vi "Vision Processing old.vi"(5 "IP Addr":string="USB 0", 7 "LED Color":T3={"Hue"={35.13837107340087, 168.7186808723669}, "Sat"={139.64285714285714, 255.0}, "Val"={145.71428571428572, 255.0}} {"Hue" scale=0.0..255.0 scale format="%#_3g"}, 8 "error in (no error)":errorcluster, 11 "Image Size":T1=enum."160x120") -> ()   [LabVIEW 2015]
uses:
  Vision Support Code/Camera Types.ctl
  <vilib>/Rock Robotics/WPI/Camera/WPI_CameraImageSize.ctl
  <vilib>/Rock Robotics/WPI/Camera/WPI_CameraWhite Balance Values.ctl
  <vilib>/Rock Robotics/WPI/Camera/WPI_CameraExposure Values.ctl
  <vilib>/Rock Robotics/WPI/Camera/WPI_CameraFrameRate.ctl
  Robot Global Data.vi
  <vilib>/Rock Robotics/Network Tables/NT Write String.vi
  <vilib>/vision/NI_Vision_Development_Module.lvlib
  Vision Target Values.vi
panel:
  out "Timings":cluster{"Call Name":string, "Delta (ms)":u32}[](array[cluster])
  out "Highest Avg Score":dbl
  in  "Min Score Threshold":i32=75
  in  "Display Original":bool=TRUE
  in  "Display Mask":bool=TRUE
  out "fps":dbl
  in  "Emphasize Limit Tests":bool=TRUE
  in  "Camera Type":T2=enum."MS HD3000 square"
  in  "Aspect Fudge Factor":dbl=1.0
  in  "Score Threshold":dbl=75.0
  out "ms to process":u32
  out "Qualified Particles":i32
  # "This is only the initial camera size.\nOther camera setup is done\non the diagram. Notice it is set\nonce before the loop but can be\nupdated within the loop if needed."
  # "Instructions:\nUse LED Color to threshold and build particles. Adjust calibration if needed.\nDisplays are very useful for debugging, but will slow down execution, so you\nmay want to disable once working.\nAnnotations show the rectangle and the scores from top to bottom.\nChange camera setting on diagram."
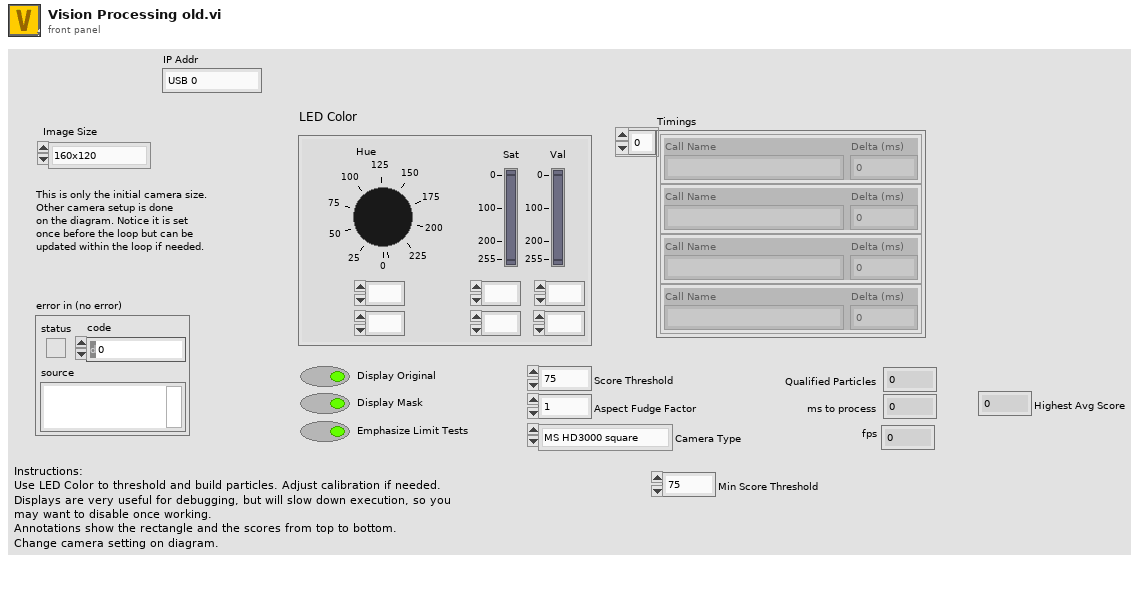
[diagram p1: front panel]
types:
  T1 = typedef "WPI_CameraImageSize.ctl" = enum16{"640x480", "320x240", "160x120", "Custom"}
  T2 = typedef "Camera Types.ctl" = enum16{"206", "1011", "1013", "MS HD3000 square", "MS HD3000 640x480"}
  T3 = cluster{"Hue":cluster{dbl, dbl}, "Sat":cluster{dbl, dbl}, "Val":cluster{dbl, dbl}}
  T4 = typedef "WPI_CameraFrameRate.ctl" = u32
  T5 = typedef "WPI_CameraExposure Values.ctl" = enum16{"Auto", "Flicker-free 50 Hz", "Flicker-free 60 Hz", "Hold current", "Custom"}
  T6 = typedef "WPI_CameraWhite Balance Values.ctl" = enum16{"Auto", "Fixed indoor", "Fixed outdoor 1", "Fixed outdoor 2", "Fixed fluorescent 1", "Fixed fluorescent 2", "Hold current", "Custom"}
  T7 = typedef "Image Type" = u32
  T8 = typedef "Particle Parameters" = i32
  T9 = typedef "WPI_CameraDevRef.ctl" = cluster{"Camera Address":string, "CameraStatus":errorcluster}
  T10 = typedef "IMAQ Image.ctl" = refnum<image>
  T11 = cluster{"Bounding box":cluster{"left":dbl, "top":dbl, "right":dbl, "bottom":dbl}, "Aspect Ratio":dbl, "Area to CH":dbl, "X Mask":dbl, "Y Mask":dbl, "Moment":dbl}[]
  T12 = cluster{"Distance (ft)":dbl, "Center":cluster{dbl, dbl}, "Normalized Rect":cluster{"Numeric":dbl, "Numeric 2":dbl, "Numeric 3":dbl, "Numeric 5":dbl}}[]
  T13 = cluster{"Detected Targets":cluster{"Distance (ft)":dbl, "Center":cluster{"X":dbl, "Y":dbl}, "Normalized Rect":cluster{"Numeric":dbl, "Numeric 2":dbl, "Numeric 3":dbl, "Numeric 5":dbl}}[]}
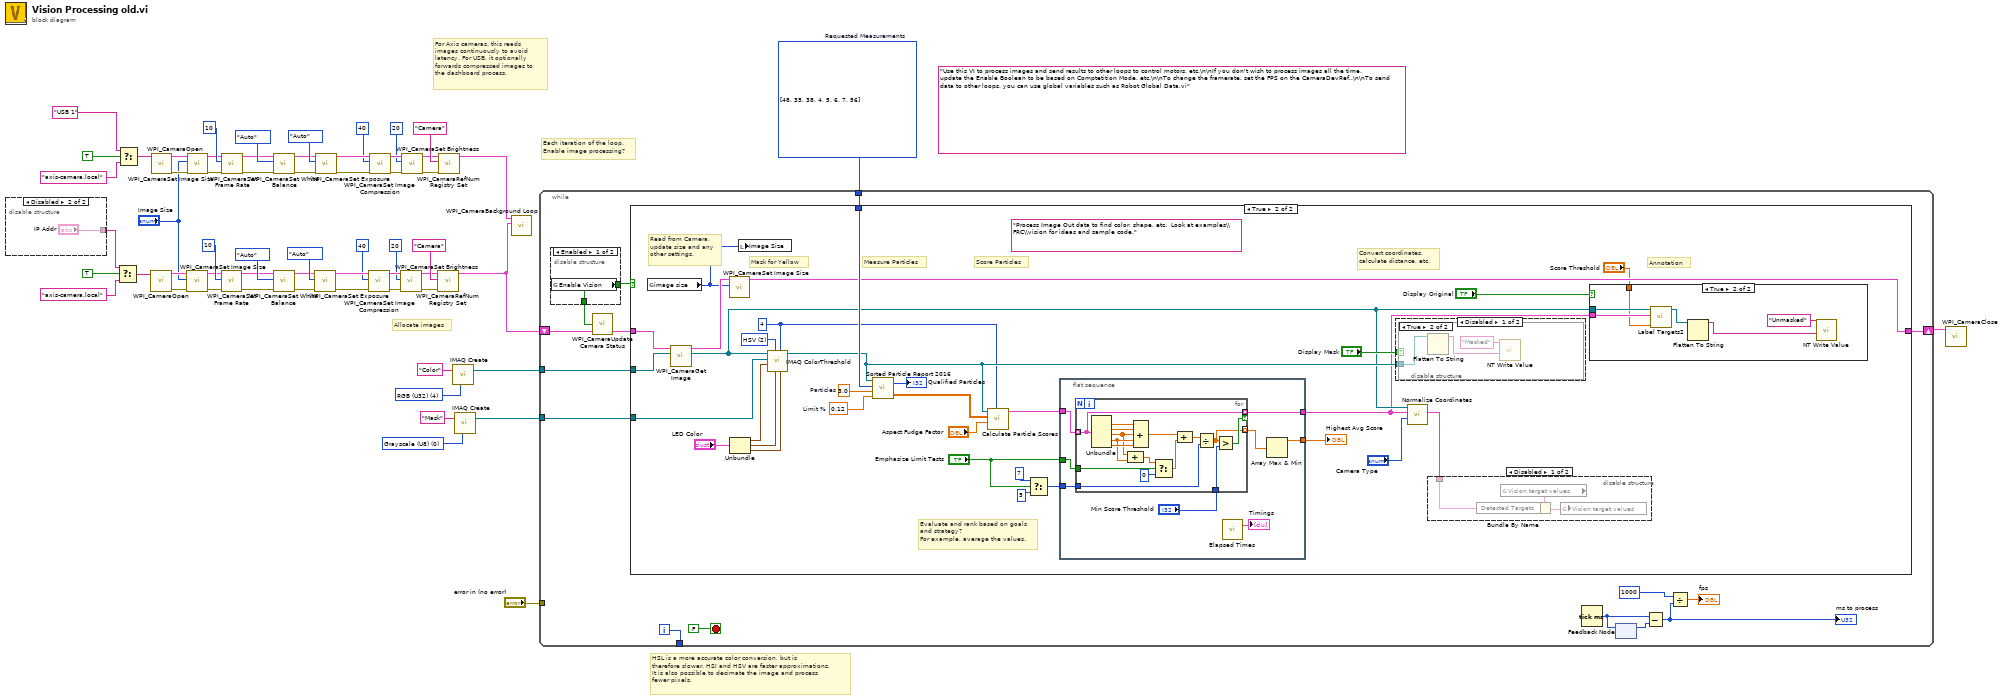
[diagram p0: block diagram]
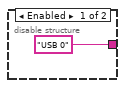
[diagram p2: hidden frame]
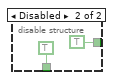
[diagram p3: hidden frame]
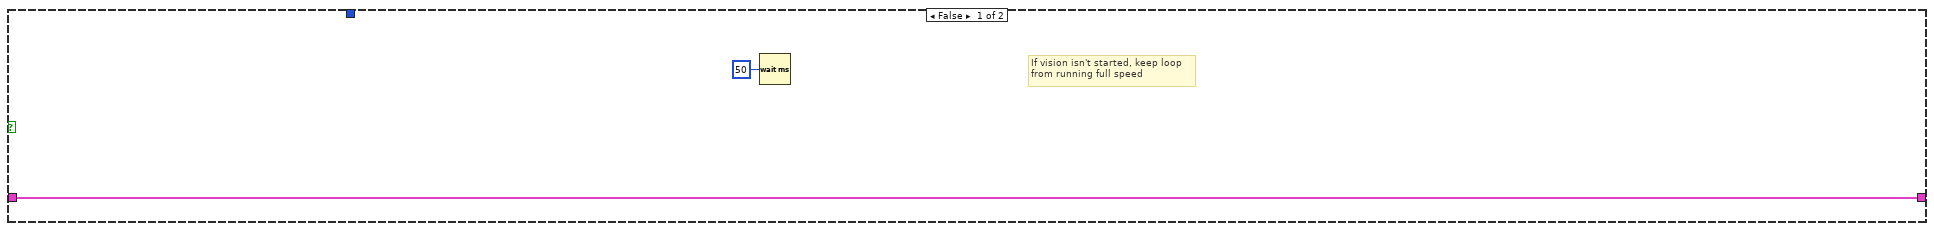
[diagram p4: hidden frame]
diagram:
  w31 = T7 0 items=["Grayscale (U8)", "Grayscale (I16)", "Grayscale (SGL)", "Complex (CSG)", "RGB (U32)", "HSL (U32)", "RGB (U64)", "Grayscale (U16)"] ("Image Type")
  w32 = T7 4 items=["Grayscale (U8)", "Grayscale (I16)", "Grayscale (SGL)", "Complex (CSG)", "RGB (U32)", "HSL (U32)", "RGB (U64)", "Grayscale (U16)"] ("Image Type")
  (unwired) "Use this VI to process images and send results to other loops to control motors, etc.\n\nIf you don't wish to process images all the time, update the Enable Boolean to be based on Comptetition Mode, etc.\n\nTo change the framerate, set the FPS on the CameraDevRef..\n\nTo send data to other loops, you can use global variables such as Robot Global Data.vi"
  w59 = T8[] [48, 35, 38, 4, 5, 6, 7, 56] items=["Center of Mass X", "Center of Mass Y", "First Pixel X", "First Pixel Y", "Bounding Rect Left", "Bounding Rect Top", "Bounding Rect Right", "Bounding Rect Bottom", "Max Feret Diameter Start X", "Max Feret Diameter Start Y", "Max Feret Diameter End X", "Max Feret Diameter End Y", "Max Horiz. Segment Length Left", "Max Horiz. Segment Length Right", "Max Horiz. Segment Length Row", "-", "Bounding Rect Width", "Bounding Rect Height", "Bounding Rect Diagonal", "Perimeter", "Convex Hull Perimeter", "Holes' Perimeter", "Max Feret Diameter", "Equivalent Ellipse Major Axis", "Equivalent Ellipse Minor Axis", "Equivalent Ellipse Minor Axis (Feret)", "Equivalent Rect Long Side", "Equivalent Rect Short Side", "Equivalent Rect Diagonal", "Equivalent Rect Short Side (Feret)", "Average Horiz. Segment Length", "Average Vert. Segment Length", "Hydraulic Radius", "Waddel Disk Diameter", "-", "Area", "Holes' Area", "Particle & Holes' Area", "Convex Hull Area", "Image Area", "-", "Number of Holes", "Number of Horiz. Segments", "Number of Vert. Segments", "-", "Orientation", "Max Feret Diameter Orientation", "-", "% Area/Image Area", "% Area/(Particle & Holes' Area)", "Ratio of Equivalent Ellipse Axes", "Ratio of Equivalent Rect Sides", "-", "Elongation Factor", "Compactness Factor", "Heywood Circularity Factor", "Type Factor", "-", "Sum X", "Sum Y", "Sum XX", "Sum XY", "Sum YY", "Sum XXX", "Sum XXY", "Sum XYY", "Sum YYY", "-", "Moment of Inertia XX", "Moment of Inertia XY", "Moment of Inertia YY", "Moment of Inertia XXX", "Moment of Inertia XXY", "Moment of Inertia XYY", "Moment of Inertia YYY", "Norm. Moment of Inertia XX", "Norm. Moment of Inertia XY", "Norm. Moment of Inertia YY", "Norm. Moment of Inertia XXX", "Norm. Moment of Inertia XXY", "Norm. Moment of Inertia XYY", "Norm. Moment of Inertia YYY", "Hu Moment 1", "Hu Moment 2", "Hu Moment 3", "Hu Moment 4", "Hu Moment 5", "Hu Moment 6", "Hu Moment 7"]  # Requested Measurements
  # "Each iteration of the loop,\nEnable image processing?"
  # "HSL is a more accurate color conversion, but is\ntherefore slower. HSI and HSV are faster approximations.\nIt is also possible to decimate the image and process\nfewer pixels."
  # "For Axis cameras, this reads\nimages continuously to avoid\nlatency. For USB, it optionally\nforwards compressed images to\nthe dashboard process."
  # "Allocate images"
  n1 = disable-structure shown="Disabled" {
    disable-tunnel: ["USB 0" ("format string") "IP Addr"] -> w56
    frame Enabled {
    }
    frame Disabled {
    }
  }
  n2 = Select(t=w56, s=TRUE ("dot notation? (F)"), f="axis-camera.local" ("format string")) -> (s? t:f=w58:string)
  n3 = Select(t="USB 1" ("format string"), s=TRUE ("dot notation? (F)"), f="axis-camera.local" ("format string")) -> (s? t:f=w27:string)
  n4 = call <vilib>:"WPI_CameraOpen.vi"("Camera Address"=w58) -> ("error out"=w47:errorcluster, "CameraDevRef"=w46:T9)  [unwired: 2 in, 7 out]
  n5 = call <vilib>:"WPI_CameraOpen.vi"("Camera Address"=w27) -> ("error out"=w17:errorcluster, "CameraDevRef"=w16:T9)  [unwired: 2 in, 7 out]
  n6 = call <vilib>:"WPI_CameraSet Image Size.vi"("error in (no error)"=w47, "Image Size"="Image Size", "CameraDevRef"=w46) -> ("error out"=w48:errorcluster, "CameraDevRef Out"=w45:T9)  [unwired: 1 in, 6 out]
  n7 = call <vilib>:"WPI_CameraSet Image Size.vi"("error in (no error)"=w17, "Image Size"="Image Size", "CameraDevRef"=w16) -> ("error out"=w18:errorcluster, "CameraDevRef Out"=w15:T9)  [unwired: 1 in, 6 out]
  n8 = call <vilib>:"WPI_CameraSet Frame Rate.vi"("error in (no error)"=w48, "Frame Rate (fps)"=T4 10, "CameraDevRef"=w45) -> ("error out"=w49:errorcluster, "CameraDevRef Out"=w44:T9)  [unwired: 7 out]
  n9 = call <vilib>:"WPI_CameraSet Frame Rate.vi"("error in (no error)"=w18, "Frame Rate (fps)"=T4 10, "CameraDevRef"=w15) -> ("error out"=w19:errorcluster, "CameraDevRef Out"=w14:T9)  [unwired: 7 out]
  n10 = call <vilib>:"WPI_CameraSet White Balance.vi"("error in (no error)"=w49, "White Balance"=WPI_CameraWhite_Balance_Values."Auto", "CameraDevRef"=w44) -> ("error out"=w29:errorcluster, "CameraDevRef Out"=w28:T9)  [unwired: 1 in, 6 out]
  n11 = call <vilib>:"WPI_CameraSet White Balance.vi"("error in (no error)"=w19, "White Balance"=WPI_CameraWhite_Balance_Values."Auto", "CameraDevRef"=w14) -> ("error out"=w6:errorcluster, "CameraDevRef Out"=w5:T9)  [unwired: 1 in, 6 out]
  n12 = call <vilib>:"WPI_CameraSet Exposure.vi"("error in (no error)"=w29, "Exposure"=WPI_CameraExposure_Values."Auto", "CameraDevRef"=w28) -> ("error out"=w50:errorcluster, "CameraDevRef Out"=w42:T9)  [unwired: 1 in, 6 out]
  n13 = call <vilib>:"WPI_CameraSet Exposure.vi"("error in (no error)"=w6, "Exposure"=WPI_CameraExposure_Values."Auto", "CameraDevRef"=w5) -> ("error out"=w20:errorcluster, "CameraDevRef Out"=w12:T9)  [unwired: 1 in, 6 out]
  n14 = call <vilib>:"WPI_CameraSet Image Compression.vi"("error in (no error)"=w50, "Compression"=40, "CameraDevRef"=w42) -> ("error out"=w51:errorcluster, "CameraDevRef Out"=w43:T9)  [unwired: 7 out]
  n15 = call <vilib>:"WPI_CameraSet Image Compression.vi"("error in (no error)"=w20, "Compression"=40, "CameraDevRef"=w12) -> ("error out"=w21:errorcluster, "CameraDevRef Out"=w13:T9)  [unwired: 7 out]
  n16 = call <vilib>:"WPI_CameraSet Brightness.vi"("error in (no error)"=w51, "Brightness"=20, "CameraDevRef"=w43) -> ("error out"=w52:errorcluster, "CameraDevRef Out"=w35:T9)  [unwired: 7 out]
  n17 = call <vilib>:"WPI_CameraSet Brightness.vi"("error in (no error)"=w21, "Brightness"=20, "CameraDevRef"=w13) -> ("error out"=w22:errorcluster, "CameraDevRef Out"=w7:T9)  [unwired: 7 out]
  n18 = call <vilib>:"WPI_CameraRefNum Registry Set.vi"("error in (no error)"=w52, "refnum name"="Camera", "CameraDevRef"=w35) -> ("CameraDevRef"=w1:T9)  [unwired: 1 in, 7 out]
  n19 = call <vilib>:"WPI_CameraRefNum Registry Set.vi"("error in (no error)"=w22, "refnum name"="Camera", "CameraDevRef"=w7) -> ("CameraDevRef"=w2:T9)  [unwired: 1 in, 7 out]
  n20 = call "IMAQ Create"("Image Name"="Color", "Image Type"=w32) -> ("New Image"=w60:T10)  [unwired: 2 in, 2 out]
  n21 = call "IMAQ Create"("Image Name"="Mask", "Image Type"=w31) -> ("New Image"=w34:T10)  [unwired: 2 in, 2 out]
  n22 = call <vilib>:"WPI_CameraBackground Loop.vi"("CameraDevRef 2"=w1, "CameraDevRef"=w2) -> ()  [unwired: 10 in]
  n23 = while {
    tunnel: w60 -> [w71]
    tunnel: w34 -> [w75]
    tunnel: w59 -> [w74]
    tunnel: "error in (no error)" -> [_]
    tunnel: [w70] -> _
    shift-right: [w66] -> w36
    shift-left: w1 -> [w68]
    i -> [w70]
    stop <- FALSE stop-if-true
    n24 = disable-structure shown="Enabled" {
      disable-tunnel: [w77 TRUE ("Enable Vision")] -> w69
      disable-tunnel: [w77 TRUE ("Enable Vision")] -> _
      frame Enabled {
        n25 = global read "Robot Global Data.vi" "Enable Vision"() -> (w77:bool)
      }
      frame Disabled {
      }
    }
    n26 = call <vilib>:"WPI_CameraUpdate Camera Status.vi"("CameraDevRef In"=w68, "Enable Vision"=w69) -> ("CameraDevRef Out"=w67:T9)  [unwired: 3 in]
    n27 = case shown="True" w69 {
      tunnel: w75 -> [_ w113]
      tunnel: w74 -> [_ w108]
      tunnel: w67 -> [w80 w104]
      tunnel: w71 -> [_ w103]
      tunnel: [w80 w101] -> w66
      frame False {
        # "If vision isn't started, keep loop\nfrom running full speed"
        n28 = Wait (ms)(milliseconds to wait=u32 50) -> ()  [unwired: 1 out]
      }
      frame True {
        w85 = 4 ("Replace Value")
        w98 = u16 2 items=["RGB", "HSL", "HSV", "HSI"] ("Color Mode")
        (unwired) "Process Image Out data to find color, shape, etc.  Look at examples\\FRC\\vision for ideas and sample code."
        w105 = 0.12  # Limit %
        w107 = 3.0  # Particles
        # "Evaluate and rank based on goals\nand strategy?\nFor example, average the values."
        # "Read from Camera,\nupdate size and any\nother settings."
        # "Measure Particles"
        # "Convert coordinates,\ncalculate distance, etc."
        # "Annotation"
        # "Score Particles"
        # "Mask for Yellow"
        n29 = global read "Robot Global Data.vi" "image size"() -> (w84:T1)
        n30 = call <vilib>:"WPI_CameraGet Image.vi"("Image"=w103, "CameraDevRef"=w104) -> ("Image Out"=w88:T10, "CameraDevRef Out"=w102:T9)  [unwired: 7 in, 1 out]
        n31 = call <vilib>:"WPI_CameraSet Image Size.vi"("Image Size"=w84, "CameraDevRef"=w102) -> ("CameraDevRef Out"=w101:T9)  [unwired: 2 in, 7 out]
        n32 = Unbundle("LED Color") -> ("Hue"=w112:cluster{dbl, dbl}, "Sat"=w111:cluster{dbl, dbl}, "Val"=w110:cluster{dbl, dbl})
        n33 = local write "Image Size"(w84) -> ()
        n34 = call "IMAQ ColorThreshold"("Blue or Luma or Val or Inten Range"=w110, "Replace Value"=w85, "Green or Sat Range"=w111, "Color Mode"=w98, "Red or Hue Range"=w112, "Image Dst"=w113, "Image Src"=w88) -> ("Image Dst Out"=w97:T10)  [unwired: 3 in, 1 out]
        n35 = call "Sorted Particle Report 2016.vi"("Min Area Size %"=w105, "Particle Count Limit"=w107, "Pixel Measurements"=w108, "Image in"=w97) -> ("Sorted Data"=w96:dbl[][], "Particles"=→"Qualified Particles":i32)
        n36 = call "Calculate Particle Scores.vi"("Pixel Value"=w85, "Aspect Fudge Factor"="Aspect Fudge Factor", "Sorted Data"=w96, "Image in"=w97) -> ("Scores"=w94:T11)  [unwired: 7 in]
        n37 = Select(t=7, s="Emphasize Limit Tests", f=5) -> (s? t:f=w91:i32)
        n38 = flat-sequence {
          tunnel: w94 -> [w134]
          tunnel: w91 -> [w132]
          tunnel: [w135] -> w90
          tunnel: [w129] -> w87
          tunnel: "Emphasize Limit Tests" -> [w133]
          frame #0 {
            n39 = for {
              tunnel: w134 -> [w149] mode=indexing
              tunnel: [w149] -> w129 mode=indexing if=w148
              tunnel: [w147] -> w130 mode=indexing
              tunnel: w132 -> [w146]
              tunnel: "Min Score Threshold" -> [w145]
              tunnel: w133 -> [w138]
              n40 = Unbundle(w149) -> ("Aspect Ratio"=w151:dbl, "Area to CH"=w150:dbl, "X Mask"=w140:dbl, "Y Mask"=w141:dbl, "Moment"=w142:dbl)  [unwired: 1 out]
              n41 = Compound Arithmetic op=ADD(w140, w141) -> (w139:dbl)
              n42 = Compound Arithmetic op=ADD(w151, w150, w140, w141, w142) -> (w144:dbl)
              n43 = Select(t=w139, s=w138, f=0) -> (s? t:f=w137:dbl)
              n44 = Compound Arithmetic op=ADD(w144, w137) -> (w143:dbl)
              n45 = Divide(x=w143, y=w146) -> (x/y=w147:dbl)
              n46 = Greater?(x=w147, y=w145) -> (0:w148:bool)
            }
            n47 = call "Elapsed Times.vi"() -> ("Timings"=→"Timings":cluster{"Call Name":string, "Delta (ms)":u32}[])  [unwired: 3 in]
            n48 = Array Max & Min(array=w130) -> (max value=w135:dbl)  [unwired: 3 out]
          }
        }
        n49 = disable-structure shown="Disabled" {
          disable-tunnel: "Display Mask" -> [w115 _]
          disable-tunnel: w97 -> [w114 _]
          frame Disabled {
            n50 = case shown="True" w115 {
              tunnel: w114 -> [_ w118]
              frame False {
              }
              frame True {
                n51 = Flatten To String(anything=w118) -> (data string=w117:string)  [unwired: 3 in, 2 out]
                n52 = call-poly <vilib>:"NT Write Value.vi"("String"=w117, "Name"="Masked") -> ()  [unwired: 9 in, 1 out]
              }
            }
          }
          frame Enabled {
          }
        }
        n53 = call "Normalize Coordinates.vi"("Camera Type"="Camera Type", "Targets"=w87, "Image in"=w88) -> ("Found Targets"=w82:T12)  [unwired: 7 in, 1 out]
        n54 = disable-structure shown="Disabled" {
          disable-tunnel: w82 -> [w119 _]
          frame Disabled {
            n55 = global read "Vision Target Values.vi" "Vision target values"() -> (w121:T13)
            n56 = Bundle By Name(cluster=w121, "Detected Targets"=w119) -> (w120:T13)
            n57 = global write "Vision Target Values.vi" "Vision target values"(w120) -> ()
          }
          frame Enabled {
          }
        }
        n58 = case shown="True" "Display Original" {
          tunnel: w88 -> [_ w127]
          tunnel: w87 -> [_ w126]
          tunnel: "Score Threshold" -> [_ w125]
          frame False {
          }
          frame True {
            n59 = call "Label Targets2.vi"("Score Threshold"=w125, "Targets"=w126, "Image in"=w127) -> ("Image out"=w124:T10)  [unwired: 8 in]
            n60 = Flatten To String(anything=w124) -> (data string=w123:string)  [unwired: 3 in, 2 out]
            n61 = call-poly <vilib>:"NT Write Value.vi"("String"=w123, "Name"="Unmasked") -> ()  [unwired: 9 in, 1 out]
          }
        }
        "Highest Avg Score" <- w90
      }
    }
    n62 = Tick Count (ms)() -> (millisecond timer value=w72:u32)
    n63 = feedback-in #1(w72) -> ()
    n64 = feedback #1() -> (w73:u32)  [unwired: 1 in]
    n65 = Subtract(x=w72, y=w73) -> (x-y=w63:u32)
    "ms to process" <- w63
    n66 = Divide(x=1000 ("Brightness"), y=w63) -> (x/y=→"fps":dbl)
  }
  n67 = call <vilib>:"WPI_CameraClose.vi"("CameraDevRef"=w36) -> ()  [unwired: 1 in, 10 out]
